vi "Module Loop.vi"(8 "error in (no error)":errorcluster, 11 "Historian Charting Manager in":refnum<class "Historian Charting Manager.lvclass">) -> (0 "error out":errorcluster, 3 "Historian Charting Manager out":refnum<class "Historian Charting Manager.lvclass">)   [LabVIEW 2020, in "VolatusGUI.lvlib" / "Historian Charting Manager.lvclass"]
uses:
  Historian Charting Manager.lvclass
  C:/dev/lv20CE/relink/lv-volatus/Volatus/Module/Module.lvclass
  Volatus/Module/Module.lvclass/Module.ctl
  Volatus/MessageQ/MessageQ.lvclass/MessageQ.ctl
  Charting Config Value/Charting Config Value.lvclass
  Duplicate Group.ctl
  Volatus/Module/Module.lvclass
  Historian Charting Manager.lvclass/Historian Charting Manager.ctl
  JSON Charting Config.ctl
  JSON Chart Group.ctl
  JSON Plot Group.ctl
  JSON Plot Config.ctl
  New Plot Group Data.ctl
  VolatusConfig/VolatusConfigElement/VolatusConfigElement.lvclass
  Chart Info.ctl
  Volatus/MessageQ/MessageQ.lvclass
  Select Plot Group Data.ctl
  Plot Group Config.ctl
  X-Axis Type.ctl
  Plot Config.ctl
  Scale.ctl
  Chart Selection.ctl
  Chart Registration.ctl
  Plot Group Events Value/Plot Group Events Value.lvclass/Plot Group Events Value.ctl
  Plot Group Removed Data.ctl
  VolatusHistorian/Historian Identity/Historian Identity.lvclass
  C:/dev/lv20CE/relink/lv-volatus/Volatus/Identity/Identity.lvclass
  PluginGUI/PluginGUI.lvclass
  Chart GUI.vi
  <vilib>/Utility/error.llb/Error Cluster From Error Code.vi
  lv-promises/Promises/Promise/Promise.lvclass
  Plot Group Events Value/Plot Group Events Value.lvclass
  GUI Helper/GUI Helper.lvclass
  Volatus/Volatus.lvlib
  Volatus/VolatusAPI/VolatusAPI.lvclass
  VolatusGUI.lvlib
panel:
  out "Cover":string
  in  "Export":bool
  in  "Import":bool
  in  "New Chart":bool
  in  "Remove Group":bool
  in  "Dup Group":bool
  in  "New Group":bool
  in  "Chart Group":string(combo)
  # "To configure channels to plot, create a chart and then use the Config button in the upper right of the new chart window to create a plot group."
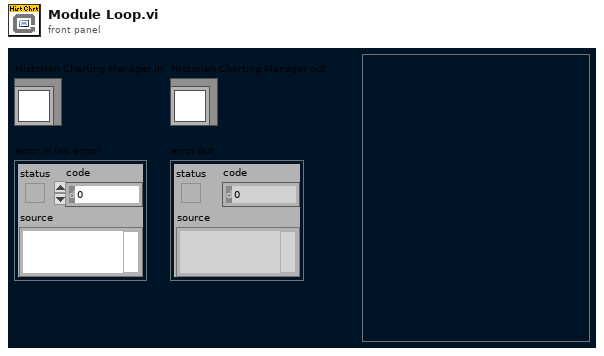
[diagram p1: front panel]
types:
  T1 = typedef "VolatusGUI.lvlib/Historian Charting Manager.lvclass/Duplicate Group.ctl" = cluster{"From":string, "Name":string}
  T2 = typedef "VolatusGUI.lvlib/JSON Charting Config.ctl" = cluster{"ChartGroups":T3[], "PlotGroups":T4[]}
  T3 = typedef "VolatusGUI.lvlib/JSON Chart Group.ctl" = cluster{"Name":string, "PlotGroups":string[]}
  T4 = typedef "VolatusGUI.lvlib/JSON Plot Group.ctl" = cluster{"Name":string, "Chart":cluster{"X-Axis":string, "X-Channel":string, "Now":bool, "Time":string, "SwapAxes":bool}, "Plots":T5[]}
  T5 = typedef "VolatusGUI.lvlib/JSON Plot Config.ctl" = cluster{"Channel":string, "Visible":bool, "Color":string, "Scale":string}
  T6 = enum32{"Invalid", "Standard", "Closed", "Hidden", "Minimized", "Maximized"}
  T7 = enum8{"Enabled", "Disabled", "Disabled and Grayed Out"}
  T8 = typedef "VolatusGUI.lvlib/Historian Charting Manager.lvclass/New Plot Group Data.ctl" = cluster{"Name":string, "Plot Groups":string[]}
  T9 = typedef "VolatusGUI.lvlib/Historian Charting Manager.lvclass/Chart Info.ctl" = cluster{"PluginGUI":refnum<class "MessageQ.lvclass">, "Select Plot Group":refnum<user-event>}
  T10 = typedef "VolatusGUI.lvlib/Historian Charting Manager.lvclass/Select Plot Group Data.ctl" = cluster{"Chart Num":i32, "Plots Config":T11, "Plot Groups":string[]}
  T11 = typedef "VolatusGUI.lvlib/Historian Charting Manager.lvclass/Plot Group Config.ctl" = cluster{"Name":string, "X-Axis Type":T12, "X-Axis Channel":string, "Plots":T13[], "Lock Now":bool, "Time":string, "Swap Axes":bool}
  T12 = typedef "VolatusGUI.lvlib/Historian Charting Manager.lvclass/X-Axis Type.ctl" = enum16{"Time", "Channel"}
  T13 = typedef "VolatusGUI.lvlib/Historian Charting Manager.lvclass/Plot Config.ctl" = cluster{"Channel":string, "Visible":bool, "Color":u32, "Scale":T14}
  T14 = typedef "VolatusGUI.lvlib/Historian Charting Manager.lvclass/Scale.ctl" = enum16{"Left", "Right"}
  T15 = typedef "VolatusGUI.lvlib/Historian Charting Manager.lvclass/Chart Selection.ctl" = cluster{"Chart Num":i32, "Plot Group":string}
  T16 = typedef "VolatusGUI.lvlib/Historian Charting Manager.lvclass/Chart Registration.ctl" = cluster{"Chart Num":i32, "Select Plot Group":refnum<user-event>}
  T17 = typedef "VolatusGUI.lvlib/Historian Charting Manager.lvclass/Plot Group Removed Data.ctl" = cluster{"Name":string, "Plot Groups":string[]}
  T18 = typedef "VolatusGUI.lvlib/Historian Charting Manager.lvclass/Plot Group Events.ctl" = cluster{"Changed":refnum<user-event>, "Removed":refnum<user-event>, "New":refnum<user-event>, "Select":refnum<user-event>}
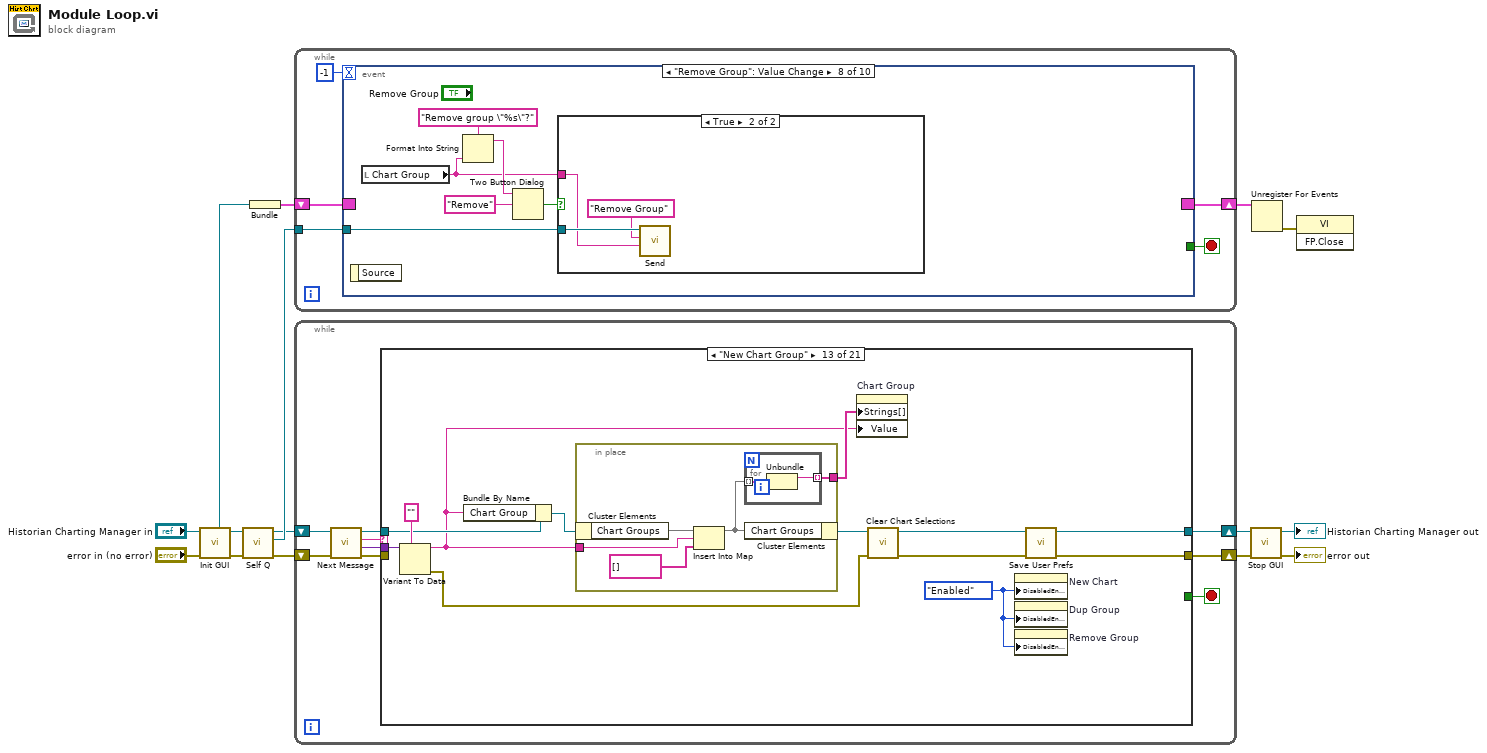
[diagram p0: block diagram]
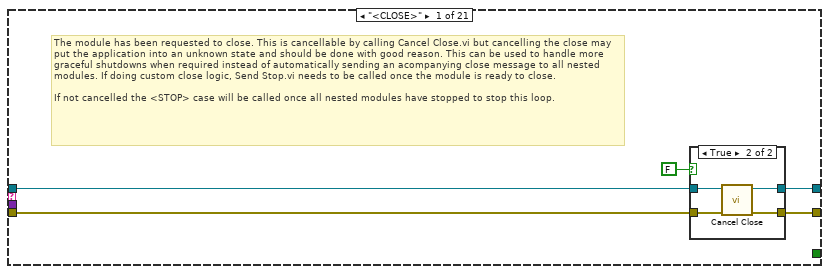
[diagram p2: hidden frame]
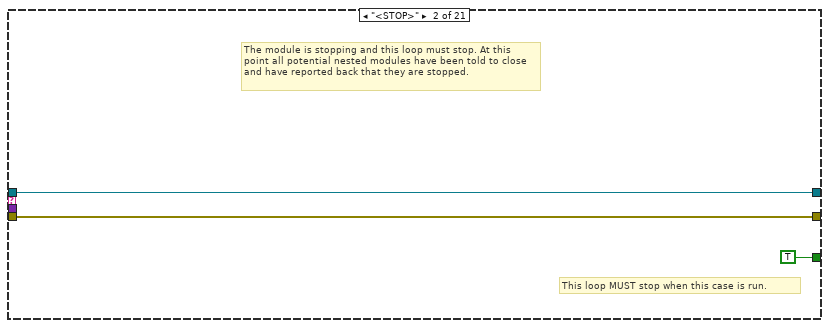
[diagram p4: hidden frame]
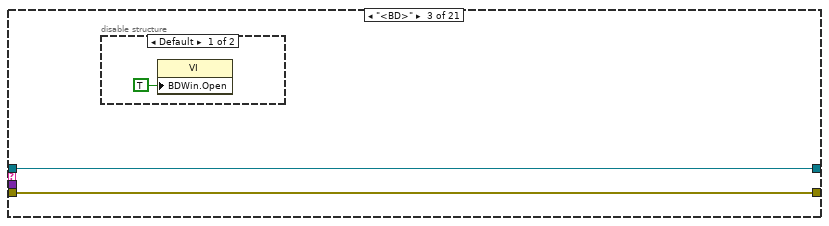
[diagram p5: hidden frame]
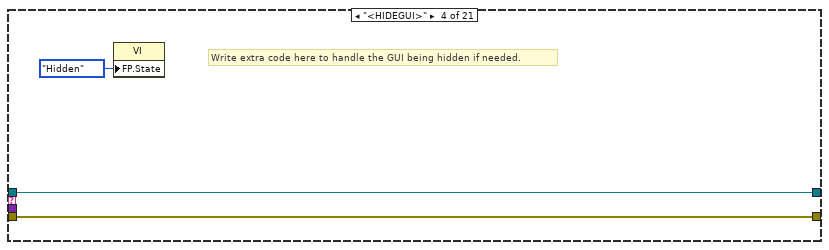
[diagram p7: hidden frame]
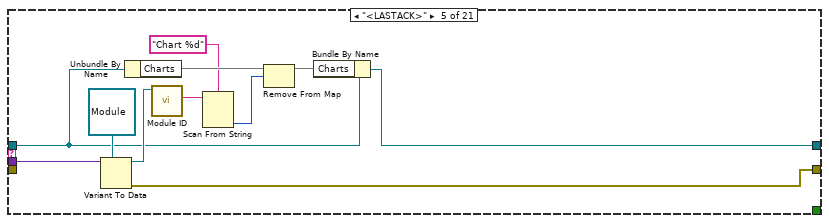
[diagram p8: hidden frame]
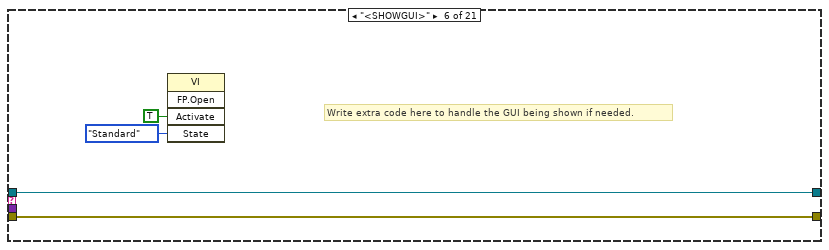
[diagram p9: hidden frame]
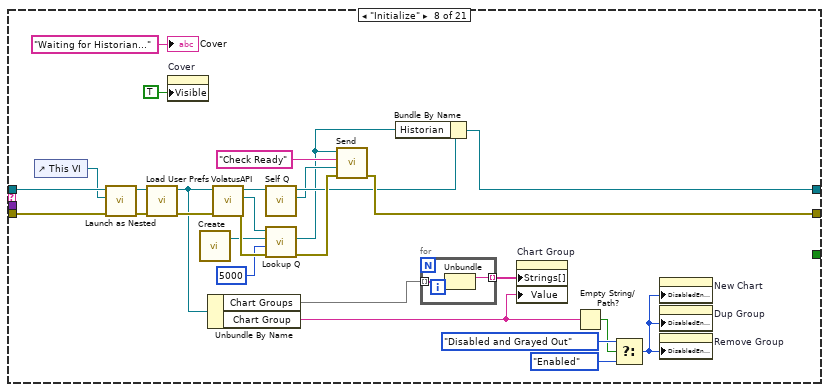
[diagram p11: hidden frame]
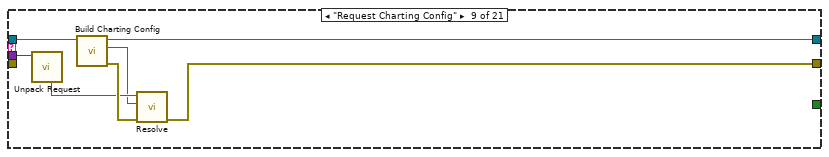
[diagram p12: hidden frame]
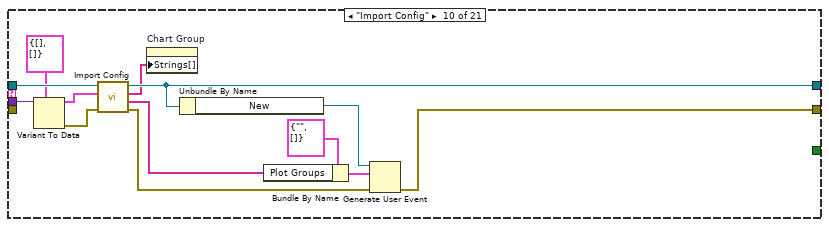
[diagram p13: hidden frame]
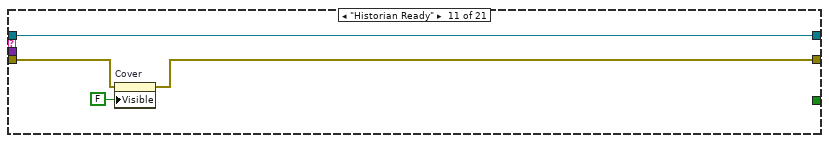
[diagram p14: hidden frame]
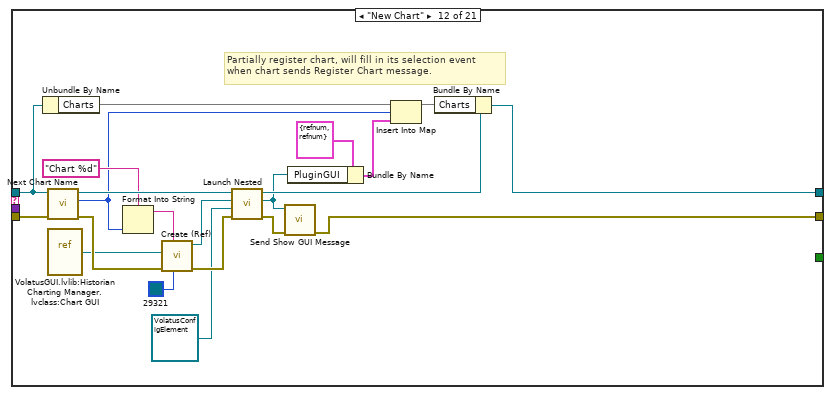
[diagram p15: hidden frame]
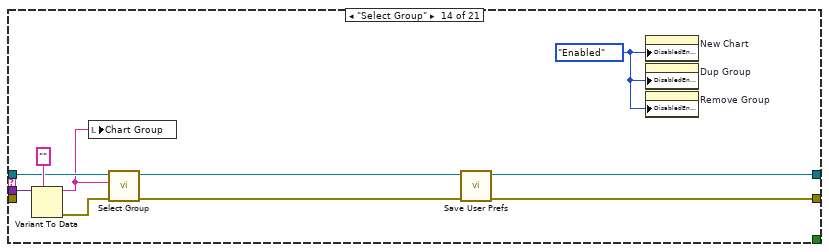
[diagram p16: hidden frame]
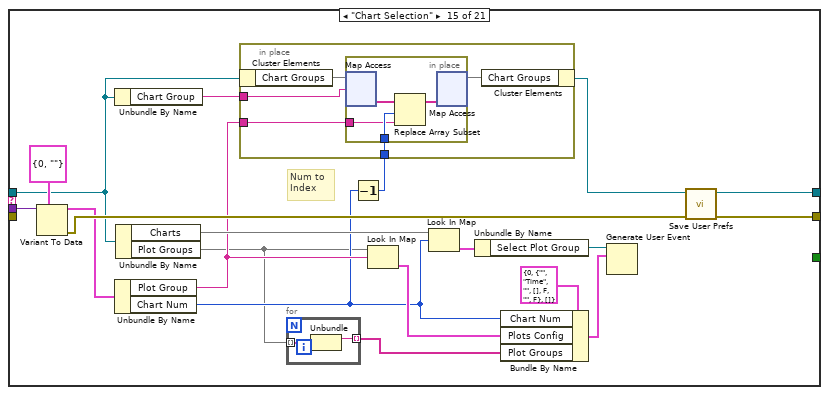
[diagram p17: hidden frame]
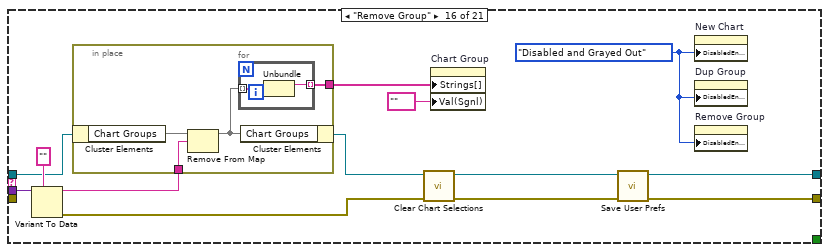
[diagram p18: hidden frame]
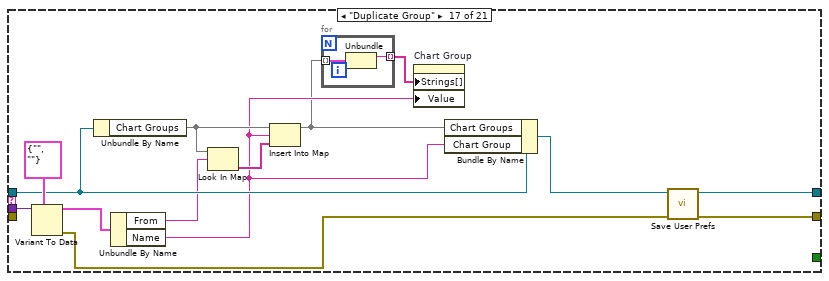
[diagram p19: hidden frame]
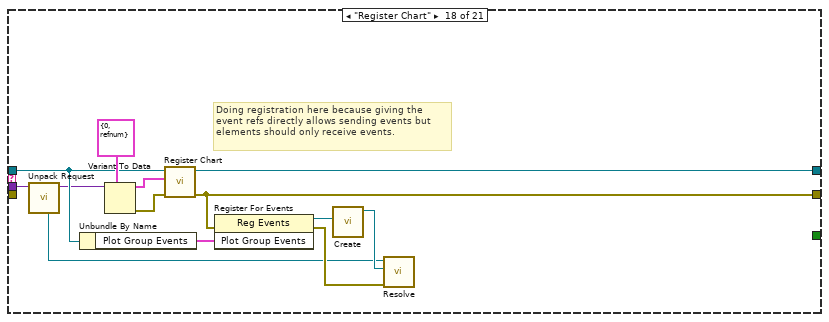
[diagram p20: hidden frame]
diagram:
  n1 = call "Init GUI.vi"("Module in"="Historian Charting Manager in") -> ("Module out"=w7:refnum<class "Historian Charting Manager.lvclass">, "Event Reg"=w12:refnum<event-registration>)  [unwired: 9 in]
  n2 = call "Self Q.vi"("Module in"=w7) -> ("Self Q"=w6:refnum<class "MessageQ.lvclass">, "Module out"=w5:refnum<class "Historian Charting Manager.lvclass">)  [unwired: 9 in]
  n3 = Bundle("Event Reg"=w12) -> (w8:cluster{"Event Reg":refnum<event-registration>})  [unwired: 1 in]
  n4 = while {
    tunnel: w6 -> [w18]
    shift-right: [w16] -> w9
    shift-left: w8 -> [w17]
    stop <- w15 stop-if-true
    n5 = event shown="[7] \"Remove Group\": Value Change" {
      selector: w17 -> [_ _ _ _ _ _ _ _ _ _]
      dyn-events: [_ _ _ _ _ _ _ _ _ _] -> w16
      timeout: -1 -> [_ _ _ _ _ _ _ _ _ _]
      tunnel: w18 -> [_ _ w22 w23 w30 w34 w44 w54 w63 w65]
      tunnel: [_ TRUE _ _ _ _ _ _ _ _] -> w15
      event Timeout {
        n6 = event-data() -> ()  [unwired: 1 in, 1 out]
      }
      event User Event {
        n7 = event-data() -> ()  [unwired: 1 in, 1 out]
      }
      event "Chart Group": Value Change {
        n8 = event-data() -> ("NewVal"=w21:string)  [unwired: 1 in]
        n9 = call "Send.vi"("Data"=w21, "ID"="Select Group", "MessageQ in"=w22) -> ()  [unwired: 7 in, 2 out]
      }
      event "Import": Value Change {
        # "Doing the prompt UI stuff here to allow other messages to still be handled by the QMH loop."
        n10 = event-data() -> ()  [unwired: 1 in, 1 out]
        n11 = call "Import Config UI.vi"() -> ("Config"=w24:T2, "Cancelled"=w25:bool)  [unwired: 10 in]
        n12 = case shown="False" w25 {
          tunnel: w24 -> [w27 _]
          tunnel: w23 -> [w28 _]
          frame False {
            n13 = call "Send.vi"("Data"=w27, "ID"="Import Config", "MessageQ in"=w28) -> ()  [unwired: 7 in, 2 out]
          }
          frame True {
          }
        }
      }
      event "Export": Value Change {
        n14 = event-data() -> ()  [unwired: 1 in, 1 out]
        n15 = call "Request.vi"("Response Type (None)"=refnum<class "Charting Config Value.lvclass"> refnum ("VolatusGUI:Charting Config Value.lvclass"), "ID"="Request Charting Config", "MessageQ in"=w30) -> ("Response"=w31:refnum<class "Charting Config Value.lvclass">)  [unwired: 6 in, 2 out]
        n16 = call "Read.vi"("Charting Config Value in"=w31) -> ("JSON Charting Config"=w29:T2)  [unwired: 10 in]
        n17 = call "Export Config UI.vi"("Config"=w29) -> ()  [unwired: 11 in]
      }
      event "New Group": Value Change {
        n18 = event-data() -> ()  [unwired: 1 in, 1 out]
        n19 = call "Group Name Prompt.vi"("Prompt"="Enter name for new group:") -> ("Cancelled"=w36:bool, "Name"=w35:string)  [unwired: 9 in]
        n20 = case shown="False" w36 {
          tunnel: w35 -> [w38 _]
          tunnel: w34 -> [w40 _]
          frame False {
            n21 = call "Send.vi"("Data"=w38, "ID"="New Chart Group", "MessageQ in"=w40) -> ()  [unwired: 7 in, 2 out]
          }
          frame True {
          }
        }
      }
      event "Dup Group": Value Change {
        n22 = event-data() -> ()  [unwired: 1 in, 1 out]
        n23 = local read "Chart Group"() -> (w42:string)
        n24 = Format Into String(format string="Enter new name for duplicated \"%s\" group:", w42) -> (resulting string=w41:string)  [unwired: 2 in, 1 out]
        n25 = call "Group Name Prompt.vi"("Prompt"=w41) -> ("Cancelled"=w45:bool, "Name"=w46:string)  [unwired: 9 in]
        n26 = case shown="False" w45 {
          tunnel: w46 -> [w50 _]
          tunnel: w44 -> [w49 _]
          tunnel: w42 -> [w51 _]
          frame False {
            n27 = Bundle By Name(cluster=T1 {"From"="", "Name"=""} ("Duplicate Group"), "From"=w51, "Name"=w50) -> (w48:T1)
            n28 = call "Send.vi"("Data"=w48, "ID"="Duplicate Group", "MessageQ in"=w49) -> ()  [unwired: 7 in, 2 out]
          }
          frame True {
          }
        }
      }
      event "Remove Group": Value Change {
        n29 = event-data() -> ()  [unwired: 1 in, 1 out]
        n30 = local read "Chart Group"() -> (w53:string)
        n31 = Format Into String(format string="Remove group \"%s\"?", w53) -> (resulting string=w56:string)  [unwired: 2 in, 1 out]
        n32 = Two Button Dialog(message=w56, 2:"Remove" ("T button name (\"OK\")")) -> (T button?=w55:bool)  [unwired: 1 in]
        n33 = case shown="True" w55 {
          tunnel: w54 -> [_ w61]
          tunnel: w53 -> [_ w59]
          frame False {
          }
          frame True {
            n34 = call "Send.vi"("Data"=w59, "ID"="Remove Group", "MessageQ in"=w61) -> ()  [unwired: 7 in, 2 out]
          }
        }
      }
      event "New Chart": Value Change {
        n35 = event-data() -> ()  [unwired: 1 in, 1 out]
        n36 = call "Send.vi"("ID"="New Chart", "MessageQ in"=w63) -> ()  [unwired: 8 in, 2 out]
      }
      event Panel Close? {
        n37 = event-data() -> ()  [unwired: 1 in, 1 out]
        n38 = call "Send.vi"("ID"="<HIDEGUI>", "MessageQ in"=w65) -> ()  [unwired: 8 in, 2 out]
        n39 = event-data("Discard?"=TRUE) -> ()  [unwired: 1 in, 1 out]
      }
    }
  }
  n40 = while {
    shift-right: [w70] -> w10
    shift-left: w5 -> [w75]
    shift-right: [w67] -> w11
    shift-left: "error in (no error)" -> [w74]
    stop <- w69 stop-if-true
    n41 = call "Next Message.vi"("error in (no error)"=w74, "Module in"=w75) -> ("error out"=w73:errorcluster, "Data"=w68:variant, "ID"=w72:string, "Module out"=w71:refnum<class "Historian Charting Manager.lvclass">)  [unwired: 6 in]
    n42 = case shown="\"New Chart Group\"" w72 {
      tunnel: w73 -> [w78 w88 w90 w94 _ w109 w111 w136 _ _ w163 w184 _ _ _ _ _ _ _ _ w326]
      tunnel: w71 -> [w79 w89 w91 w95 w101 w110 w112 w134 w146 w161 w165 w173 w196 w211 w222 w257 w278 w286 w304 w314 w324]
      tunnel: [w77 w89 w91 w95 w99 w110 w112 w116 w145 w156 w165 w170 w188 w207 w218 w249 w269 w291 w296 w306 w323] -> w70
      tunnel: [_ TRUE _ _ _ _ _ _ _ _ _ _ _ _ _ _ _ _ _ _ _] -> w69
      tunnel: w68 -> [_ _ _ _ w106 _ _ _ w147 w160 _ _ w199 w216 w235 w260 w280 w287 w303 w316 _]
      tunnel: [w76 w88 w90 w94 w104 w109 w111 w137 w142 w149 w162 w177 w190 w209 w217 w251 w267 w283 w298 w307 w325] -> w67
      frame "<CLOSE>" {
        # "The module has been requested to close. This is cancellable by calling Cancel Close.vi but cancelling the close may put the application into an unknown state and should be done with good reason. This can be used to handle more graceful shutdowns when required instead of automatically sending an acompanying close message to all nested modules. If doing custom close logic, Send Stop.vi needs to be called once the module is ready to close.\n\nIf not cancelled the <STOP> case will be called once all nested modules have stopped to stop this loop."
        n43 = case shown="True" FALSE {
          tunnel: w78 -> [w81 w86]
          tunnel: [w81 w85] -> w76
          tunnel: w79 -> [w82 w84]
          tunnel: [w82 w83] -> w77
          frame False {
          }
          frame True {
            n44 = call "Cancel Close.vi"("error in (no error)"=w86, "Module in"=w84) -> ("error out"=w85:errorcluster, "Module out"=w83:refnum<class "Historian Charting Manager.lvclass">)  [unwired: 8 in]
          }
        }
      }
      frame "<STOP>" {
        # "This loop MUST stop when this case is run."
        # "The module is stopping and this loop must stop. At this point all potential nested modules have been told to close and have reported back that they are stopped."
      }
      frame "<BD>" {
        n45 = disable-structure shown="Default" {
          frame condition #0 (active) {
            n46 = property class="VI"("BDWin.Open"=TRUE ("Block Diagram Window:Open")) -> ()  [unwired: 2 in, 2 out]
          }
          frame condition #1 {
          }
        }
      }
      frame "<HIDEGUI>" {
        # "Write extra code here to handle the GUI being hidden if needed."
        n47 = property class="VI"("FP.State"=T6."Hidden" ("Front Panel Window:State")) -> ()  [unwired: 2 in, 2 out]
      }
      frame "<LASTACK>" {
        n48 = Variant To Data(type=refnum<class "Module.lvclass"> refnum ("Volatus:Module"), Variant=w106) -> (data=w103:refnum<class "Module.lvclass">, error out=w104:errorcluster)  [unwired: 1 in]
        n49 = Unbundle By Name(w101) -> ("Charts"=w102:map{i32, T9})
        n50 = call-dynamic "Module ID.vi"("Module in"=w103) -> ("Module ID"=w98:string)  [unwired: 10 in]
        n51 = Scan From String(format string="Chart %d", input string=w98) -> (output 1=w96:i32)  [unwired: 3 in, 3 out]
        n52 = Remove From Map(10:w96, 11:w102) -> (3:w100:map{i32, T9})  [unwired: 2 out]
        n53 = Bundle By Name(cluster=w101, "Charts"=w100) -> (w99:refnum<class "Historian Charting Manager.lvclass">)
      }
      frame "<SHOWGUI>" {
        # "Write extra code here to handle the GUI being shown if needed."
        n54 = invoke class="VI" method="FP.Open"("Activate"=TRUE ("Activate?"), "State"=T6."Standard") -> ()  [unwired: 3 in, 5 out]
      }
      frame "<TIMEOUT>" {
        # "No message for this module was received in time"
      }
      frame "Initialize" {
        n55 = control-ref of="This VI"() -> (w133:refnum<vi>)
        n56 = call "Launch as Nested.vi"("error in (no error)"=w136, "GUI"=w133, "Parent in"=w134) -> ("error out"=w135:errorcluster, "Parent"=w132:refnum<class "Historian Charting Manager.lvclass">)  [unwired: 6 in, 1 out]
        n57 = call "Load User Prefs.vi"("error in (no error)"=w135, "Historian Charting Manager in"=w132) -> ("error out"=w138:errorcluster, "Historian Charting Manager out"=w125:refnum<class "Historian Charting Manager.lvclass">)  [unwired: 8 in]
        n58 = property on="Cover" class="Str"("Visible"=TRUE) -> ()  [unwired: 2 in, 2 out]
        n59 = call "Create.vi"() -> ("Historian Identity out"=w119:refnum<class "Historian Identity.lvclass">)  [unwired: 7 in]
        n60 = Unbundle By Name(w125) -> ("Chart Groups"=w131:map{string, string[]}, "Chart Group"=w127:string)
        n61 = call "VolatusAPI.vi"("Module in"=w125) -> ("VolatusAPI"=w117:refnum<class "VolatusAPI.lvclass">, "Module out"=w118:refnum<class "Historian Charting Manager.lvclass">)  [unwired: 9 in]
        n62 = call "Self Q.vi"("Module in"=w118) -> ("Self Q"=w123:refnum<class "MessageQ.lvclass">, "Module out"=w124:refnum<class "Historian Charting Manager.lvclass">)  [unwired: 9 in]
        n63 = call "Lookup Q.vi"("error in (no error)"=w138, "Timeout ms (0)"=5000, "Identity"=w119, "VolatusAPI in"=w117) -> ("error out"=w139:errorcluster, "MessageQ"=w115:refnum<class "MessageQ.lvclass">)  [unwired: 5 in, 1 out]
        n64 = call "Send.vi"("error in (no error)"=w139, "Data"=w123, "ID"="Check Ready", "MessageQ in"=w115) -> ("error out"=w137:errorcluster)  [unwired: 6 in, 1 out]
        n65 = Bundle By Name(cluster=w124, "Historian"=w115) -> (w116:refnum<class "Historian Charting Manager.lvclass">)
        n66 = for {
          tunnel: w131 -> [w141] mode=indexing
          tunnel: [w140] -> w130 mode=indexing
          n67 = Unbundle(w141) -> ("Chart Group"=w140:string)  [unwired: 1 out]
        }
        n68 = property on="Chart Group" class="CmbBox"("Strings[]"=w130, "Value"=w127) -> ()  [unwired: 2 in, 2 out]
        n69 = Empty String/Path?(string/path=w127) -> (empty?=w126:bool)
        n70 = Select(t=T7."Disabled and Grayed Out" ("Disabled"), s=w126, f=T7."Enabled") -> (s? t:f=w113:T7)
        n71 = property on="New Chart" class="Bool"("DisabledEnum"=w113) -> ()  [unwired: 2 in, 2 out]
        n72 = property on="Dup Group" class="Bool"("DisabledEnum"=w113) -> ()  [unwired: 2 in, 2 out]
        n73 = property on="Remove Group" class="Bool"("DisabledEnum"=w113) -> ()  [unwired: 2 in, 2 out]
        "Cover" <- "Waiting for Historian..." ("Cover")
      }
      frame "Request Charting Config" {
        n74 = call "Unpack Request.vi"("Request Data"=w147) -> ("Promise"=w144:refnum<class "Promise.lvclass">)  [unwired: 8 in, 2 out]
        n75 = call "Build Charting Config.vi"("Historian Charting Manager in"=w146) -> ("error out"=w148:errorcluster, "Charting Config Value"=w143:refnum<class "Charting Config Value.lvclass">, "Historian Charting Manager out"=w145:refnum<class "Historian Charting Manager.lvclass">)  [unwired: 8 in]
        n76 = call "Resolve.vi"("error in (no error)"=w148, "Result (None)"=w143, "Promise in"=w144) -> ("error out"=w142:errorcluster)  [unwired: 7 in, 1 out]
      }
      frame "Import Config" {
        n77 = Variant To Data(type=T2 {"ChartGroups"=[], "PlotGroups"=[]} ("JSON Charting Config"), Variant=w160) -> (data=w158:T2, error out=w157:errorcluster)  [unwired: 1 in]
        n78 = call "Import Config.vi"("error in (no error)"=w157, "JSON Charting Config"=w158, "Historian Charting Manager in"=w161) -> ("error out"=w150:errorcluster, "Plot Groups"=w152:string[], "Chart Groups"=w151:string[], "Historian Charting Manager out"=w156:refnum<class "Historian Charting Manager.lvclass">)  [unwired: 5 in]
        n79 = property on="Chart Group" class="CmbBox"("Strings[]"=w151) -> ()  [unwired: 2 in, 2 out]
        n80 = Unbundle By Name(w156) -> ("New"=w155:refnum<user-event>)
        n81 = Bundle By Name(cluster=T8 {"Name"="", "Plot Groups"=[]} ("event data"), "Plot Groups"=w152) -> (w153:T8)
        n82 = Generate User Event(user event=w155, event data cluster=w153, error in=w150) -> (error out=w149:errorcluster)  [unwired: 1 in, 1 out]
      }
      frame "Historian Ready" {
        n83 = property on="Cover" class="Str"(error in=w163, "Visible"=FALSE) -> (error out=w162:errorcluster)  [unwired: 1 in, 1 out]
      }
      frame "New Chart" {
        # "Partially register chart, will fill in its selection event when chart sends Register Chart message."
        n84 = Unbundle By Name(w173) -> ("Charts"=w172:map{i32, T9})
        n85 = call "Next Chart Name.vi"("error in (no error)"=w184, "Historian Charting Manager in"=w173) -> ("error out"=w185:errorcluster, "Next Chart Num"=w168:i32, "Historian Charting Manager out"=w182:refnum<class "Historian Charting Manager.lvclass">)  [unwired: 7 in]
        n86 = vi-ref "VolatusGUI.lvlib:Historian Charting Manager.lvclass:Chart GUI.vi"() -> (w183:refnum<vi>)
        n87 = Format Into String(format string="Chart %d", w168) -> (resulting string=w174:string)  [unwired: 2 in, 1 out]
        n88 = call "Create (Ref).vi"("Color (Default)"=u32 29321, "Name"=w174, "error in (no error)"=w185, "VI"=w183) -> ("error out"=w186:errorcluster, "PluginGUI out"=w181:refnum<class "PluginGUI.lvclass">)  [unwired: 6 in]
        n89 = call "Launch Nested.vi"("error in (no error)"=w186, "Config Element"=refnum<class "VolatusConfigElement.lvclass"> refnum, "Nested Module"=w181, "Parent in"=w182) -> ("error out"=w178:errorcluster, "MessageQ"=w166:refnum<class "MessageQ.lvclass">, "Parent out"=w179:refnum<class "Historian Charting Manager.lvclass">)  [unwired: 5 in]
        n90 = call "Send Show GUI Message.vi"("error in (no error)"=w178, "MessageQ"=w166) -> ("error out"=w177:errorcluster)  [unwired: 9 in]
        n91 = Bundle By Name(cluster=T9 {"PluginGUI"=refnum, "Select Plot Group"=refnum} ("value"), "PluginGUI"=w166) -> (w167:T9)
        n92 = Insert Into Map(map in=w172, key=w168, value=w167) -> (map out=w169:map{i32, T9})  [unwired: 2 out]
        n93 = Bundle By Name(cluster=w179, "Charts"=w169) -> (w170:refnum<class "Historian Charting Manager.lvclass">)
      }
      frame "New Chart Group" {
        w187 = T7."Enabled" ("Disabled")
        n94 = Variant To Data(type="", Variant=w199) -> (data=w191:string, error out=w197:errorcluster)  [unwired: 1 in]
        n95 = Bundle By Name(cluster=w196, "Chart Group"=w191) -> (w192:refnum<class "Historian Charting Manager.lvclass">)
        n96 = in-place {
          in-place-border: w191 -> [w203]
          in-place-border: [w200] -> w193
          n97 = in-place-cluster #1(w192) -> ("Chart Groups"=w204:map{string, string[]})
          n98 = Insert Into Map(map in=w204, key=w203, value=string[] []) -> (map out=w201:map{string, string[]})  [unwired: 2 out]
          n99 = for {
            tunnel: w201 -> [w206] mode=indexing
            tunnel: [w205] -> w200 mode=indexing
            n100 = Unbundle(w206) -> ("Chart Group"=w205:string)  [unwired: 1 out]
          }
          n101 = in-place-cluster #1("Chart Groups"=w201) -> (w194:refnum<class "Historian Charting Manager.lvclass">)
        }
        n102 = property on="Chart Group" class="CmbBox"("Strings[]"=w193, "Value"=w191) -> ()  [unwired: 2 in, 2 out]
        n103 = call "Clear Chart Selections.vi"("error in (no error)"=w197, "Historian Charting Manager in"=w194) -> ("error out"=w195:errorcluster, "Historian Charting Manager out"=w189:refnum<class "Historian Charting Manager.lvclass">)  [unwired: 8 in]
        n104 = property on="New Chart" class="Bool"("DisabledEnum"=w187) -> ()  [unwired: 2 in, 2 out]
        n105 = property on="Dup Group" class="Bool"("DisabledEnum"=w187) -> ()  [unwired: 2 in, 2 out]
        n106 = property on="Remove Group" class="Bool"("DisabledEnum"=w187) -> ()  [unwired: 2 in, 2 out]
        n107 = call "Save User Prefs.vi"("error in (no error)"=w195, "Historian Charting Manager in"=w189) -> ("error out"=w190:errorcluster, "Historian Charting Manager out"=w188:refnum<class "Historian Charting Manager.lvclass">)  [unwired: 8 in]
      }
      frame "Select Group" {
        w214 = T7."Enabled" ("Disabled")
        n108 = Variant To Data(type="", Variant=w216) -> (data=w210:string, error out=w213:errorcluster)  [unwired: 1 in]
        n109 = local write "Chart Group"(w210) -> ()
        n110 = call "Select Group.vi"("error in (no error)"=w213, "Group (Empty = none)"=w210, "Historian Charting Manager in"=w211) -> ("error out"=w212:errorcluster, "Historian Charting Manager out"=w208:refnum<class "Historian Charting Manager.lvclass">)  [unwired: 7 in]
        n111 = call "Save User Prefs.vi"("error in (no error)"=w212, "Historian Charting Manager in"=w208) -> ("error out"=w209:errorcluster, "Historian Charting Manager out"=w207:refnum<class "Historian Charting Manager.lvclass">)  [unwired: 8 in]
        n112 = property on="New Chart" class="Bool"("DisabledEnum"=w214) -> ()  [unwired: 2 in, 2 out]
        n113 = property on="Dup Group" class="Bool"("DisabledEnum"=w214) -> ()  [unwired: 2 in, 2 out]
        n114 = property on="Remove Group" class="Bool"("DisabledEnum"=w214) -> ()  [unwired: 2 in, 2 out]
      }
      frame "Chart Selection" {
        # "Num to Index"
        n115 = Variant To Data(type=T15 {"Chart Num"=0, "Plot Group"=""} ("Chart Selection"), Variant=w235) -> (data=w233:T15, error out=w236:errorcluster)  [unwired: 1 in]
        n116 = Unbundle By Name(w222) -> ("Chart Group"=w221:string)
        n117 = Unbundle By Name(w233) -> ("Plot Group"=w224:string, "Chart Num"=w223:i32)
        n118 = Unbundle By Name(w222) -> ("Charts"=w232:map{i32, T9}, "Plot Groups"=w220:map{string, T11})
        n119 = for {
          tunnel: w220 -> [w238] mode=indexing
          tunnel: [w237] -> w219 mode=indexing
          n120 = Unbundle(w238) -> ("Name"=w237:string)  [unwired: 1 out]
        }
        n121 = Decrement(x=w223) -> (x-1=w225:i32)
        n122 = in-place {
          in-place-border: w221 -> [w242]
          in-place-border: w225 -> [w240]
          in-place-border: w224 -> [w239]
          n123 = in-place-cluster #2(w222) -> ("Chart Groups"=w243:map{string, string[]})
          n124 = in-place {
            in-place-border: w240 -> [w245]
            in-place-border: w239 -> [w244]
            n125 = in-place-map #3(w243, w242) -> (w247:string[])  [unwired: 1 in, 1 out]
            n126 = Replace Array Subset(array=w247, new element=w244, index=w245) -> (w246:string[])
            n127 = in-place-map #3(w246) -> (w241:map{string, string[]})  [unwired: 1 in, 2 out]
          }
          n128 = in-place-cluster #2("Chart Groups"=w241) -> (w226:refnum<class "Historian Charting Manager.lvclass">)
        }
        n129 = Look In Map(map=w220, key=w224) -> (value=w227:T11)  [unwired: 1 in, 1 out]
        n130 = Look In Map(map=w232, key=w223) -> (value=w231:T9)  [unwired: 1 in, 1 out]
        n131 = Unbundle By Name(w231) -> ("Select Plot Group"=w230:refnum<user-event>)
        n132 = Bundle By Name(cluster=T10 {"Chart Num"=0, "Plots Config"={"Name"="", "X-Axis Type"=enum."Time", "X-Axis Channel"="", "Plots"=[], "Lock Now"=FALSE, "Time"="", "Swap Axes"=FALSE}, "Plot Groups"=[]} ("event data"), "Chart Num"=w223, "Plots Config"=w227, "Plot Groups"=w219) -> (w228:T10)
        n133 = Generate User Event(user event=w230, event data cluster=w228) -> ()  [unwired: 2 in, 2 out]
        n134 = call "Save User Prefs.vi"("error in (no error)"=w236, "Historian Charting Manager in"=w226) -> ("error out"=w217:errorcluster, "Historian Charting Manager out"=w218:refnum<class "Historian Charting Manager.lvclass">)  [unwired: 8 in]
      }
      frame "Remove Group" {
        w258 = T7."Disabled and Grayed Out" ("Disabled")
        n135 = Variant To Data(type="", Variant=w260) -> (data=w256:string, error out=w254:errorcluster)  [unwired: 1 in]
        n136 = in-place {
          in-place-border: w256 -> [w263]
          in-place-border: [w261] -> w248
          n137 = in-place-cluster #4(w257) -> ("Chart Groups"=w264:map{string, string[]})
          n138 = Remove From Map(10:w263, 11:w264) -> (3:w262:map{string, string[]})  [unwired: 2 out]
          n139 = for {
            tunnel: w262 -> [w266] mode=indexing
            tunnel: [w265] -> w261 mode=indexing
            n140 = Unbundle(w266) -> ("Chart Group"=w265:string)  [unwired: 1 out]
          }
          n141 = in-place-cluster #4("Chart Groups"=w262) -> (w255:refnum<class "Historian Charting Manager.lvclass">)
        }
        n142 = call "Clear Chart Selections.vi"("error in (no error)"=w254, "Historian Charting Manager in"=w255) -> ("error out"=w253:errorcluster, "Historian Charting Manager out"=w250:refnum<class "Historian Charting Manager.lvclass">)  [unwired: 8 in]
        n143 = property on="Chart Group" class="CmbBox"("Strings[]"=w248, "Val(Sgnl)"="" ("Chart Group")) -> ()  [unwired: 2 in, 2 out]
        n144 = call "Save User Prefs.vi"("error in (no error)"=w253, "Historian Charting Manager in"=w250) -> ("error out"=w251:errorcluster, "Historian Charting Manager out"=w249:refnum<class "Historian Charting Manager.lvclass">)  [unwired: 8 in]
        n145 = property on="New Chart" class="Bool"("DisabledEnum"=w258) -> ()  [unwired: 2 in, 2 out]
        n146 = property on="Dup Group" class="Bool"("DisabledEnum"=w258) -> ()  [unwired: 2 in, 2 out]
        n147 = property on="Remove Group" class="Bool"("DisabledEnum"=w258) -> ()  [unwired: 2 in, 2 out]
      }
      frame "Duplicate Group" {
        n148 = Variant To Data(type=T1 {"From"="", "Name"=""} ("Duplicate Group"), Variant=w280) -> (data=w277:T1, error out=w268:errorcluster)  [unwired: 1 in]
        n149 = Unbundle By Name(w278) -> ("Chart Groups"=w275:map{string, string[]})
        n150 = Unbundle By Name(w277) -> ("From"=w276:string, "Name"=w272:string)
        n151 = Look In Map(map=w275, key=w276) -> (value=w274:string[])  [unwired: 1 in, 1 out]
        n152 = Insert Into Map(map in=w275, key=w272, value=w274) -> (map out=w271:map{string, string[]})  [unwired: 2 out]
        n153 = for {
          tunnel: w271 -> [w282] mode=indexing
          tunnel: [w281] -> w270 mode=indexing
          n154 = Unbundle(w282) -> ("Chart Group"=w281:string)  [unwired: 1 out]
        }
        n155 = property on="Chart Group" class="CmbBox"("Strings[]"=w270, "Value"=w272) -> ()  [unwired: 2 in, 2 out]
        n156 = Bundle By Name(cluster=w278, "Chart Groups"=w271, "Chart Group"=w272) -> (w273:refnum<class "Historian Charting Manager.lvclass">)
        n157 = call "Save User Prefs.vi"("error in (no error)"=w268, "Historian Charting Manager in"=w273) -> ("error out"=w267:errorcluster, "Historian Charting Manager out"=w269:refnum<class "Historian Charting Manager.lvclass">)  [unwired: 8 in]
      }
      frame "Register Chart" {
        # "Doing registration here because giving the event refs directly allows sending events but elements should only receive events."
        n158 = call "Unpack Request.vi"("Request Data"=w287) -> ("Data"=w285:variant, "Promise"=w284:refnum<class "Promise.lvclass">)  [unwired: 8 in, 1 out]
        n159 = Unbundle By Name(w286) -> ("Plot Group Events"=w289:T18)
        n160 = Variant To Data(type=T16 {"Chart Num"=0, "Select Plot Group"=refnum} ("Chart Registration"), Variant=w285) -> (data=w293:T16, error out=w292:errorcluster)  [unwired: 1 in]
        n161 = call "Register Chart.vi"("error in (no error)"=w292, "Chart Registration"=w293, "Historian Charting Manager in"=w286) -> ("error out"=w283:errorcluster, "Historian Charting Manager out"=w291:refnum<class "Historian Charting Manager.lvclass">)  [unwired: 7 in]
        n162 = register-events(error in=w283, w289) -> (reference out=w288:refnum<event-registration>, error out=w295:errorcluster)  [unwired: 1 in]
        n163 = call "Create.vi"("Plot Group"=w288) -> ("Plot Group Events Value out"=w290:refnum<class "Plot Group Events Value.lvclass">)  [unwired: 10 in]
        n164 = call "Resolve.vi"("error in (no error)"=w295, "Result (None)"=w290, "Promise in"=w284) -> ()  [unwired: 7 in, 2 out]
      }
      frame "Update Plots Config" {
        n165 = Variant To Data(type=T11 {"Name"="", "X-Axis Type"=enum."Time", "X-Axis Channel"="", "Plots"=[], "Lock Now"=FALSE, "Time"="", "Swap Axes"=FALSE} ("Plot Group Config"), Variant=w303) -> (data=w301:T11, error out=w300:errorcluster)  [unwired: 1 in]
        n166 = call "Update Plots Config.vi"("error in (no error)"=w300, "Plot Group Config"=w301, "Historian Charting Manager in"=w304) -> ("error out"=w299:errorcluster, "Historian Charting Manager out"=w297:refnum<class "Historian Charting Manager.lvclass">)  [unwired: 7 in]
        n167 = call "Save User Prefs.vi"("error in (no error)"=w299, "Historian Charting Manager in"=w297) -> ("error out"=w298:errorcluster, "Historian Charting Manager out"=w296:refnum<class "Historian Charting Manager.lvclass">)  [unwired: 8 in]
      }
      frame "Remove Plot Group" {
        n168 = Variant To Data(type="", Variant=w316) -> (data=w308:string)  [unwired: 1 in, 1 out]
        n169 = in-place {
          in-place-border: w308 -> [w319]
          in-place-border: [w317] -> w309
          n170 = in-place-cluster #5(w314) -> ("Plot Groups"=w320:map{string, T11})
          n171 = Remove From Map(10:w319, 11:w320) -> (3:w318:map{string, T11})  [unwired: 2 out]
          n172 = in-place-cluster #5("Plot Groups"=w318) -> (w305:refnum<class "Historian Charting Manager.lvclass">)
          n173 = for {
            tunnel: w318 -> [w322] mode=indexing
            tunnel: [w321] -> w317 mode=indexing
            n174 = Unbundle(w322) -> ("Name"=w321:string)  [unwired: 1 out]
          }
        }
        n175 = Bundle By Name(cluster=T17 {"Name"="", "Plot Groups"=[]} ("event data"), "Plot Groups"=w309, "Name"=w308) -> (w311:T17)
        n176 = Unbundle By Name(w305) -> ("Removed"=w313:refnum<user-event>)
        n177 = Generate User Event(user event=w313, event data cluster=w311) -> (error out=w310:errorcluster)  [unwired: 2 in, 1 out]
        n178 = call "Save User Prefs.vi"("error in (no error)"=w310, "Historian Charting Manager in"=w305) -> ("error out"=w307:errorcluster, "Historian Charting Manager out"=w306:refnum<class "Historian Charting Manager.lvclass">)  [unwired: 8 in]
      }
      frame Default {
        n179 = call "Report Unhandled Message ID.vi"("error in (no error)"=w326, "Module in"=w324) -> ("error out"=w325:errorcluster, "Module out"=w323:refnum<class "Historian Charting Manager.lvclass">)  [unwired: 8 in]
      }
    }
  }
  n180 = call "Stop GUI.vi"("error in (no error)"=w11, "Module in"=w10) -> ("error out"=→"error out":errorcluster, "Module out"=→"Historian Charting Manager out":refnum<class "Historian Charting Manager.lvclass">)  [unwired: 8 in]
  n181 = Unregister For Events(event registration refnum=w9) -> (error out=w13:errorcluster)  [unwired: 1 in]
  n182 = invoke class="VI" method="FP.Close"(error in=w13) -> ()  [unwired: 2 in, 3 out]
